vi "Panel.vi"(11 "TCPConfigPanel in":refnum<class "TCPConfigPanel.lvclass">) -> ()   [LabVIEW 2020, in "LV-Term.lvlib" / "TCPConfigPanel.lvclass"]
uses:
  TCPConfigPanel.lvclass
  TCPConfigPanel.lvclass/TCPConfigPanel.ctl
  <vilib>/IlluminatedG/IG OOPanel/OOPanel/Panel/Basic UI State.ctl
  <vilib>/IlluminatedG/IG OOPanel/OOPanel/Panel/Panel.lvclass
  <vilib>/IlluminatedG/IG OOPanel/OOPanel/OOPanel.lvlib
  C:/Program Files (x86)/National Instruments/LabVIEW 2020/vi.lib/IlluminatedG/IG OOPanel/OOPanel/Panel/Panel.lvclass
  C:/dev/illuminated-g/lv-terminal-app/LV-Term/TCPConfigPanel/TCPConfigPanel.lvclass
  C:/dev/illuminated-g/lv-terminal-app/LV-Term/ConfigPanel/ConfigPanel.lvclass
panel:
  in  "Port":u16
  in  "Hostname / IP":string
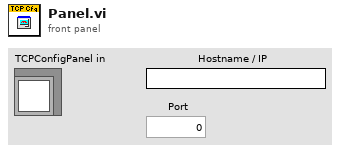
[diagram p1: front panel]
types:
  T1 = typedef "OOPanel.lvlib/Panel.lvclass/Basic UI State.ctl" = enum16{"Init", "Run", "Close"}
  T2 = typedef "OOPanel.lvlib/Panel.lvclass/Panel Events.ctl" = cluster{"Visbility":refnum<user-event>, "Close":refnum<user-event>}
  T3 = typedef "LV-Term.lvlib/TCPConfigPanel.lvclass/Ref Data.ctl" = cluster{"Host":string, "Port":u16}
  T4 = typedef "OOPanel.lvlib/Panel.lvclass/Visibility State.ctl" = enum16{"Idle", "Closed", "Hidden", "Visible", "Subpanel"}
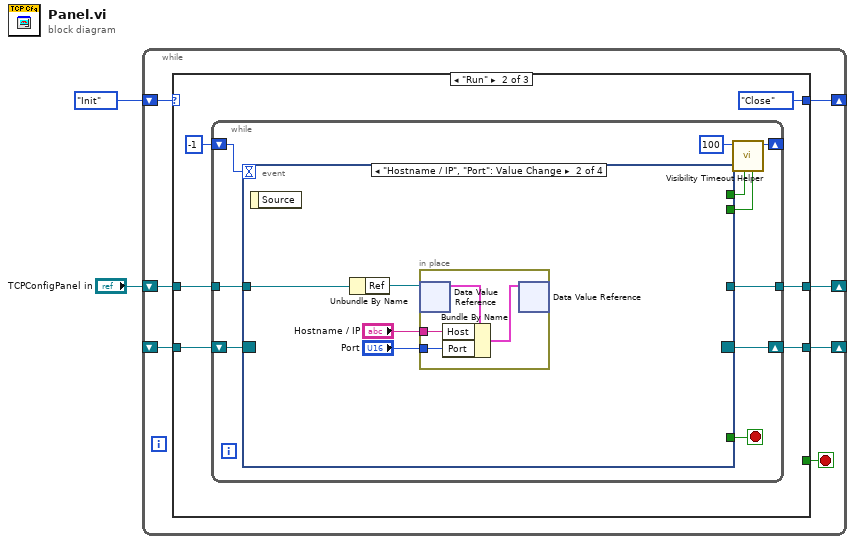
[diagram p0: block diagram]
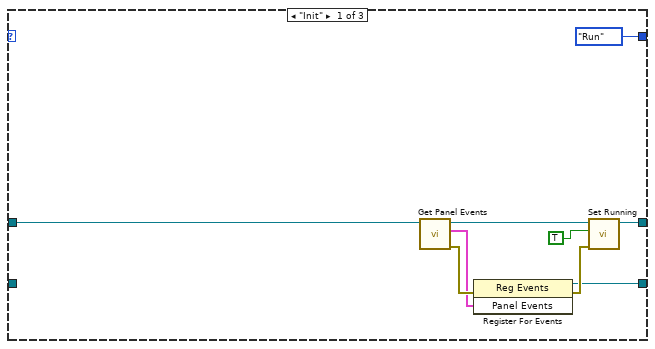
[diagram p2: hidden frame]
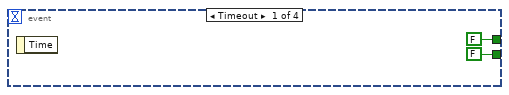
[diagram p3: hidden frame]
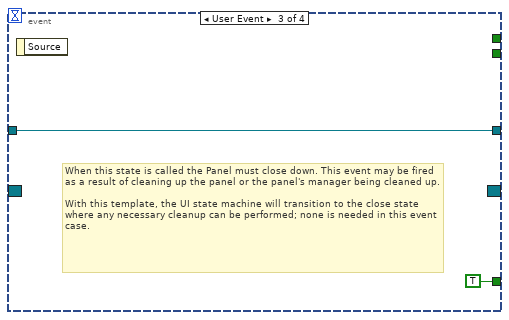
[diagram p4: hidden frame]
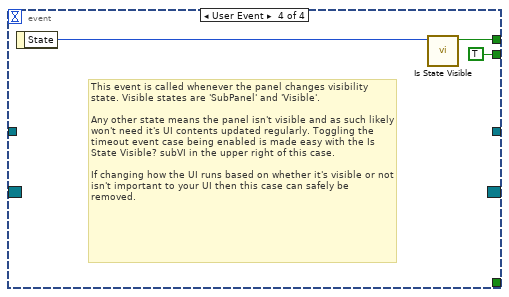
[diagram p5: hidden frame]
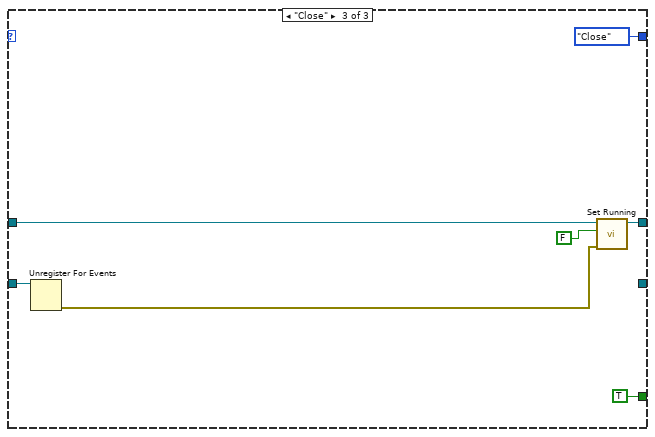
[diagram p6: hidden frame]
diagram:
  n1 = while {
    shift-right: [w8] -> _
    shift-left: _ -> [w9]
    shift-right: [w6] -> _
    shift-left: Basic_UI_State."Init" ("Basic UI State") -> [w7]
    shift-right: [w4] -> _
    shift-left: "TCPConfigPanel in" -> [w3]
    stop <- w5 stop-if-true
    n2 = case shown="\"Run\"" w7 {
      tunnel: w9 -> [_ w24 w52]
      tunnel: [w12 w22 _] -> w8
      tunnel: [Basic_UI_State."Run" ("Basic UI State") Basic_UI_State."Close" ("Basic UI State") Basic_UI_State."Close" ("Basic UI State")] -> w6
      tunnel: [_ _ TRUE] -> w5
      tunnel: [w11 w19 w50] -> w4
      tunnel: w3 -> [w10 w20 w51]
      frame "Init" {
        n3 = call <vilib>:"Get Panel Events.vi"("Panel in"=w10) -> ("error out"=w18:errorcluster, "Panel Events"=w14:T2, "Panel out"=w15:refnum<class "TCPConfigPanel.lvclass">)  [unwired: 8 in]
        n4 = register-events(error in=w18, w14) -> (reference out=w12:refnum<event-registration>, error out=w16:errorcluster)  [unwired: 1 in]
        n5 = call <vilib>:"Set Running.vi"("error in (no error)"=w16, "Running"=TRUE, "Panel in"=w15) -> ("Panel out"=w11:refnum<class "TCPConfigPanel.lvclass">)  [unwired: 7 in, 1 out]
      }
      frame "Run" {
        n6 = while {
          shift-right: [w30] -> w22
          shift-left: w24 -> [w31]
          shift-right: [w33] -> _
          shift-left: -1 ("Timeout") -> [w32]
          tunnel: w20 -> [w26]
          tunnel: [w25] -> w19
          stop <- w27 stop-if-true
          n7 = event shown="[1] \"Hostname / IP\", \"Port\": Value Change" {
            selector: w31 -> [_ _ _ _]
            dyn-events: [_ _ _ _] -> w30
            timeout: w32 -> [_ _ _ _]
            tunnel: [FALSE _ _ w48] -> w29
            tunnel: [FALSE _ _ TRUE] -> w28
            tunnel: [_ _ TRUE _] -> w27
            tunnel: w26 -> [_ w39 w45 _]
            tunnel: [_ _ w45 _] -> w25
            event Timeout {
              n8 = event-data() -> ()  [unwired: 1 in, 1 out]
            }
            event "Hostname / IP", "Port": Value Change {
              n9 = event-data() -> ()  [unwired: 1 in, 1 out]
              n10 = Unbundle By Name(w39) -> ("Ref"=w40:refnum<data-value>)
              n11 = in-place {
                in-place-border: "Hostname / IP" -> [w42]
                in-place-border: "Port" -> [w41]
                n12 = in-place-dvr #1(w40) -> (w44:T3)  [unwired: 1 out]
                n13 = Bundle By Name(cluster=w44, "Host"=w42, "Port"=w41) -> (w43:T3)
                n14 = in-place-dvr #1(w43) -> ()  [unwired: 2 out]
              }
            }
            event User Event {
              # "When this state is called the Panel must close down. This event may be fired as a result of cleaning up the panel or the panel's manager being cleaned up.\n\nWith this template, the UI state machine will transition to the close state where any necessary cleanup can be performed; none is needed in this event case."
              n15 = event-data() -> ()  [unwired: 1 in, 1 out]
            }
            event User Event {
              # "This event is called whenever the panel changes visibility state. Visible states are 'SubPanel' and 'Visible'.\n\nAny other state means the panel isn't visible and as such likely won't need it's UI contents updated regularly. Toggling the timeout event case being enabled is made easy with the Is State Visible? subVI in the upper right of this case.\n\nIf changing how the UI runs based on whether it's visible or not isn't important to your UI then this case can safely be removed."
              n16 = event-data() -> ("State"=w49:T4)  [unwired: 1 in]
              n17 = call <vilib>:"Is State Visible.vi"("Visibility"=w49) -> ("Visible"=w48:bool)  [unwired: 10 in]
            }
          }
          n18 = call <vilib>:"Visibility Timeout Helper.vi"("Update?"=w28, "Use Timeout?"=w29, "Visible Timeout mS"=100) -> ("Timeout"=w33:i32)  [unwired: 8 in]
        }
      }
      frame "Close" {
        n19 = Unregister For Events(event registration refnum=w52) -> (error out=w54:errorcluster)  [unwired: 1 in]
        n20 = call <vilib>:"Set Running.vi"("error in (no error)"=w54, "Running"=FALSE, "Panel in"=w51) -> ("Panel out"=w50:refnum<class "TCPConfigPanel.lvclass">)  [unwired: 7 in, 1 out]
      }
    }
  }
